vi "ADS1015 Init.vi"(7 "I2C Channel":u8=1, 8 "error in (no error)":errorcluster, 9 "ADS1015 Config Options":T1={"I2C"={"Slave Address"=72, "Channel"=1}, "ADC"={"Channel"=4, "Expected Range (Programmable Gain Amplifier)"=0, "Sampling Mode"=1, "Sampling Rate"=4, "Comparator Mode"=1, "Comparator Polarity"=1, "Latching Comparator"=1, "Comparator Queue & Disable"=3}} {"ADC"."Comparator Queue & Disable" items=["Assert after one conversion", "Assert after two conversions", "Assert after four conversions", "Comparator disabled"]; "ADC"."Latching Comparator" items=["Non-latching", "Latching"]; "ADC"."Comparator Polarity" items=["Active Low", "Active High"]; "ADC"."Comparator Mode" items=["Traditional Comparator w/ hysteresis", "Window Comparator"]; "ADC"."Sampling Rate" items=["128SPS", "250SPS", "490SPS", "920SPS", "1600SPS", "2400SPS", "3300SPS"]; "ADC"."Sampling Mode" items=["Continuous Conversion", "Single-shot (Low Power)"]; "ADC"."Expected Range (Programmable Gain Amplifier)" items=["+/-6.144V", "+/-4.096V", "+/-2.048V", "+/-1.024V", "+/-0.512V", "+/-0.256V"]; "ADC"."Channel" items=["Differential: Ch 0&1", "Differential: Ch 0&3", "Differential: Ch 1&3", "Differential: Ch 2&3", "Single Ended: Ch 0", "Single Ended: Ch 1", "Single Ended: Ch 2", "Single Ended: Ch 3"]; "I2C"."Slave Address" format="%.0x"}, 10 "I2C Slave Address":u8=72 format="%.0x", 11 "LINX Resource in":T2) -> (0 "error out":errorcluster, 1 "ADS1015 Config Options":T1={"I2C"={"Slave Address"=72, "Channel"=1}, "ADC"={"Channel"=4, "Expected Range (Programmable Gain Amplifier)"=0, "Sampling Mode"=1, "Sampling Rate"=4, "Comparator Mode"=1, "Comparator Polarity"=1, "Latching Comparator"=1, "Comparator Queue & Disable"=3}} {"ADC"."Comparator Queue & Disable" items=["Assert after one conversion", "Assert after two conversions", "Assert after four conversions", "Comparator disabled"]; "ADC"."Latching Comparator" items=["Non-latching", "Latching"]; "ADC"."Comparator Polarity" items=["Active Low", "Active High"]; "ADC"."Comparator Mode" items=["Traditional Comparator w/ hysteresis", "Window Comparator"]; "ADC"."Sampling Rate" items=["128SPS", "250SPS", "490SPS", "920SPS", "1600SPS", "2400SPS", "3300SPS"]; "ADC"."Sampling Mode" items=["Continuous Conversion", "Single-shot (Low Power)"]; "ADC"."Expected Range (Programmable Gain Amplifier)" items=["+/-6.144V", "+/-4.096V", "+/-2.048V", "+/-1.024V", "+/-0.512V", "+/-0.256V"]; "ADC"."Channel" items=["Differential: Ch 0&1", "Differential: Ch 0&3", "Differential: Ch 1&3", "Differential: Ch 2&3", "Single Ended: Ch 0", "Single Ended: Ch 1", "Single Ended: Ch 2", "Single Ended: Ch 3"]; "I2C"."Slave Address" format="%.0x"}, 3 "LINX Resource out":T2)   [LabVIEW 2014]
uses:
  <vilib>/MakerHub/LINX/Private/Type Defs/LINX Ref.ctl
  <vilib>/MakerHub/LINX/Private/Type Defs/Platform.ctl
  <vilib>/MakerHub/LINX/Private/Type Defs/Interface.ctl
  <vilib>/MakerHub/LINX/Private/Device/Type Defs/LINX Device Config.ctl
  <vilib>/MakerHub/LINX/Private/Device/Type Defs/TCP Config.ctl
  <vilib>/MakerHub/LINX/Private/Device/Type Defs/Channels.ctl
  ADS1015 Config Options.ctl
  <vilib>/MakerHub/LINX/LMH-LINX.lvlib
  <vilib>/MakerHub/LINX/Private/Device/Device.lvlib
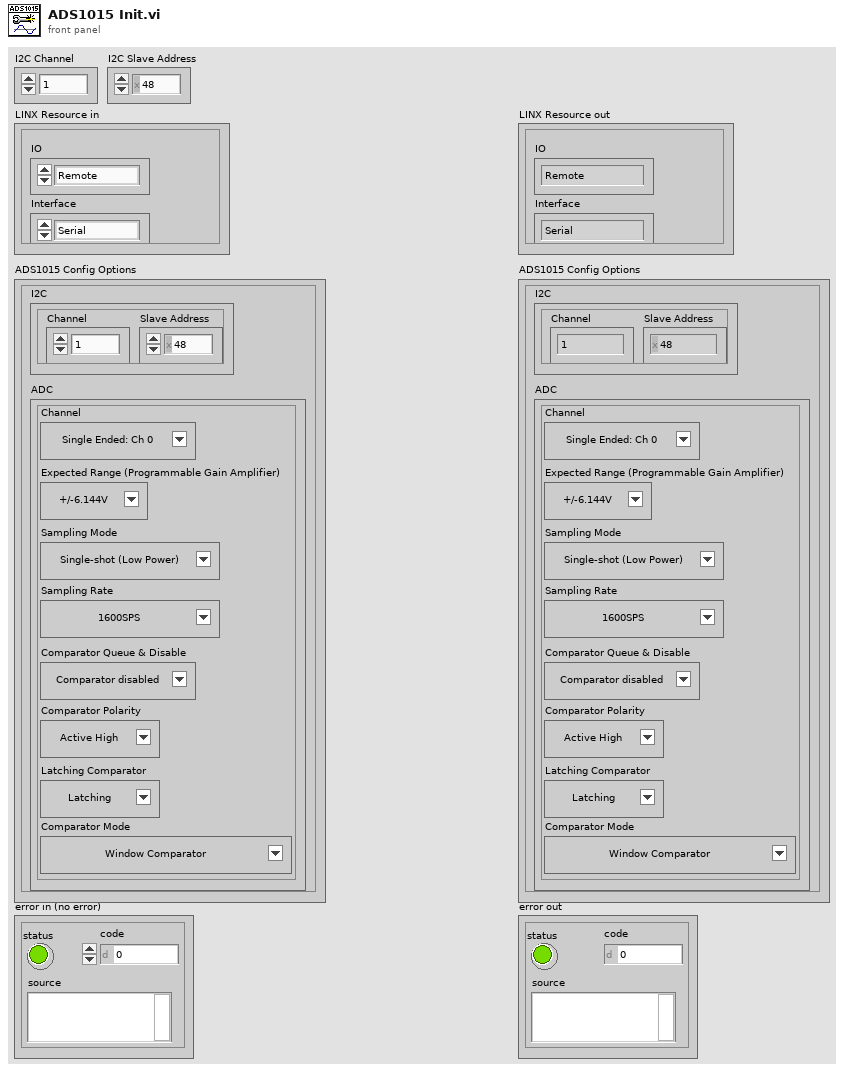
[diagram p1: front panel]
types:
  T1 = typedef "ADS1015 Config Options.ctl" = cluster{"I2C":cluster{"Slave Address":u8, "Channel":u8}, "ADC":cluster{"Channel":u8, "Expected Range (Programmable Gain Amplifier)":u8, "Sampling Mode":u8, "Sampling Rate":u8, "Comparator Mode":u8, "Comparator Polarity":u8, "Latching Comparator":u8, "Comparator Queue & Disable":u8}}
  T2 = typedef "LMH-LINX.lvlib/LINX Ref.ctl" = cluster{"IO":T3, "Interface":T4, "LINX Device Config":T5}
  T3 = typedef "LMH-LINX.lvlib/Platform.ctl" = enum16{"Remote", "Local"}
  T4 = typedef "LMH-LINX.lvlib/Interface.ctl" = enum16{"Serial", "TCP"}
  T5 = typedef "LMH-LINX.lvlib/Device.lvlib/LINX Device Config.ctl" = cluster{"Interface":T4, "COM Port":refnum<visa-resource-name>, "TCP Configuration":T6, "Device Family":u8, "Device ID":u8, "Device Name":string, "TCP Ref":refnum<k5>, "Channels":T7}
  T6 = typedef "LMH-LINX.lvlib/Device.lvlib/TCP Config.ctl" = cluster{"IP Address":string, "Port":u16}
  T7 = typedef "LMH-LINX.lvlib/Channels.ctl" = cluster{"DI":u8[], "DO":u8[], "AI":u8[], "AO":u8[], "PWM":u8[], "QE":u8[], "UART":u8[], "I2C 2":u8[], "SPI":u8[], "CAN":u8[], "Servo":u8[], "AI Ref (V)":dbl, "AI Resolution (Bits)":u8, "AO Ref (V)":dbl, "AO Resolution (Bits)":u8}
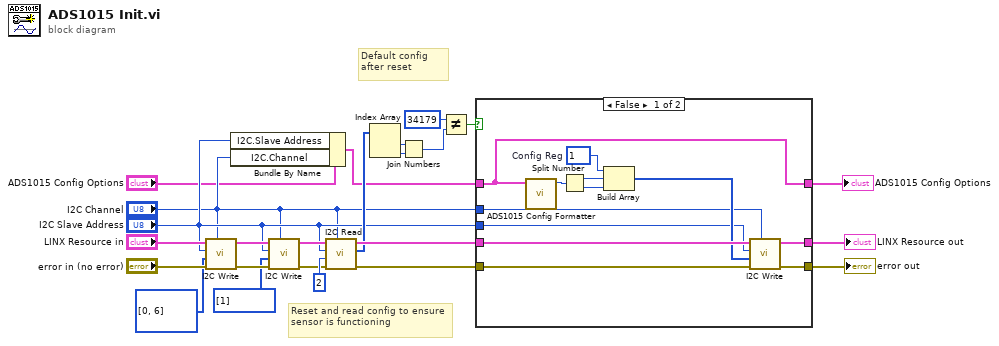
[diagram p0: block diagram]
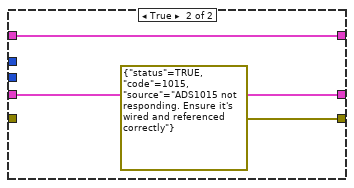
[diagram p2: hidden frame]
diagram:
  # "Default config after reset"
  # "Reset and read config to ensure sensor is functioning"
  n1 = call <vilib>:"I2C Write.vi"("I2C Channel"="I2C Channel", "Error In"="error in (no error)", "Data"=u8[] [0, 6], "I2C Slave Address (0)"="I2C Slave Address", "LINX Resource"="LINX Resource in") -> ("Error Out"=w10:errorcluster, "LINX Resource"=w9:T2)  [unwired: 5 in]
  n2 = Bundle By Name(cluster="ADS1015 Config Options", "I2C.Slave Address"="I2C Slave Address", "I2C.Channel"="I2C Channel") -> (w1:T1)
  n3 = call <vilib>:"I2C Write.vi"("I2C Channel"="I2C Channel", "Error In"=w10, "Data"=u8[] [1], "I2C Slave Address (0)"="I2C Slave Address", "LINX Resource"=w9) -> ("Error Out"=w7:errorcluster, "LINX Resource"=w8:T2)  [unwired: 5 in]
  n4 = call <vilib>:"I2C Read.vi"("I2C Channel"="I2C Channel", "Error In"=w7, "Bytes To Read"=u8 2, "I2C Slave Address (0)"="I2C Slave Address", "LINX Resource"=w8) -> ("Error Out"=w20:errorcluster, "Data"=w15:u8[], "LINX Resource"=w21:T2)  [unwired: 4 in]
  n5 = Index Array(array=w15) -> (element #1=w13:u8, element #2=w14:u8)  [unwired: 2 in]
  n6 = Join Numbers(hi=w13, lo=w14) -> ((hi.lo)=w12:u16)
  n7 = Not Equal?(x=u16 34179, y=w12) -> (x != y?=w16:bool)
  n8 = case shown="False" w16 {
    tunnel: w21 -> [w36 w39]
    tunnel: [w27 w39] -> w23
    tunnel: w20 -> [w35 _]
    tunnel: [w26 errorcluster {"status"=TRUE, "code"=1015, "source"="ADS1015 not responding. Ensure it's wired and referenced correctly"} ("error constant")] -> w22
    tunnel: "I2C Channel" -> [w29 _]
    tunnel: "I2C Slave Address" -> [w28 _]
    tunnel: w1 -> [w25 w37]
    tunnel: [w25 w37] -> w5
    frame False {
      w31 = u8 1  # Config Reg
      n9 = call "ADS1015 Config Formatter.vi"("ADS1015 Config Options"=w25) -> ("Config Command"=w34:u16)  [unwired: 10 in]
      n10 = Split Number(x=w34) -> (hi(x)=w33:u8, lo(x)=w32:u8)
      n11 = Build Array(w31, w33, w32) -> (w30:u8[])
      n12 = call <vilib>:"I2C Write.vi"("I2C Channel"=w29, "Error In"=w35, "Data"=w30, "I2C Slave Address (0)"=w28, "LINX Resource"=w36) -> ("Error Out"=w26:errorcluster, "LINX Resource"=w27:T2)  [unwired: 5 in]
    }
    frame True {
    }
  }
  "error out" <- w22
  "LINX Resource out" <- w23
  "ADS1015 Config Options" <- w5
